vi "Get Attributes.vi"(5 "Flatten Pointer?":bool, 7 "Test ID":string, 8 "error in (no error)":errorcluster, 10 "Include Private?":bool, 11 "Test Executive in":refnum<class "Test Executive.lvclass">) -> (0 "error out":errorcluster, 1 "Attributes":variant[](array[variant]), 2 "Attribute Names out":string[](array[string]), 3 "Test Executive out":refnum<class "Test Executive.lvclass">, 4 "Found?":bool, 6 "Data IDs":string[](array[string]))   [LabVIEW 2017, in "Test Executive.lvlib" / "Test Executive.lvclass"]
uses:
  <vilib>/gpm_packages/@cs/test-executive/Source/Test Executive/TestExecutive/Test Executive.lvclass
  <vilib>/gpm_packages/@cs/test-executive/Source/Test Executive/TestExecutive/Test Executive.lvclass/Test Executive.ctl
  <vilib>/gpm_packages/@cs/linked-list/Source/Linked List/Linked List Ref/Linked List Ref.lvclass
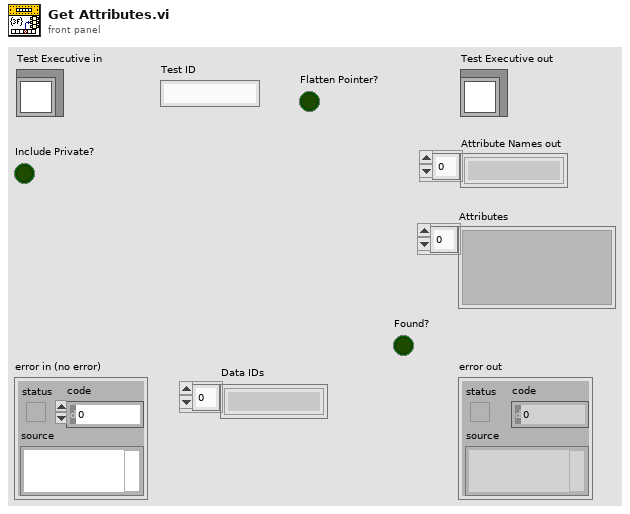
[diagram p1: front panel]
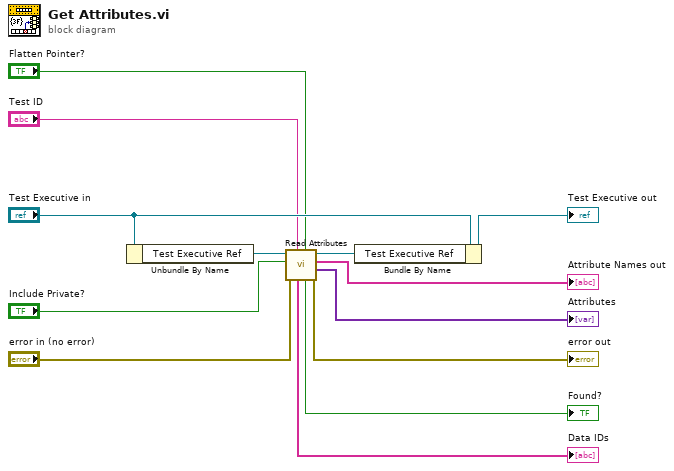
[diagram p0: block diagram]
diagram:
  n1 = Unbundle By Name("Test Executive in") -> ("Test Executive Ref"=w13:refnum<data-value>)
  n2 = call <vilib>:"Read Attributes.vi"("Flatten Pointer?"="Flatten Pointer?", "Linked List ID"="Test ID", "error in (no error)"="error in (no error)", "Include Private?"="Include Private?", "Linked List Ref"=w13) -> ("error out"=→"error out":errorcluster, "Attributes"=→"Attributes":variant[], "Attribute Names out"=→"Attribute Names out":string[], "Linked List Ref out"=w12:refnum<data-value>, "found"=→"Found?":bool, "Data IDs"=→"Data IDs":string[])  [unwired: 1 in]
  n3 = Bundle By Name(cluster="Test Executive in", "Test Executive Ref"=w12) -> (→"Test Executive out":refnum<class "Test Executive.lvclass">)
